vi "Remove newlines from comments.vi"(11 "Comments IN":string caption="Comments") -> (3 "Comments OUT":string caption="Comments")   [LabVIEW 2010]
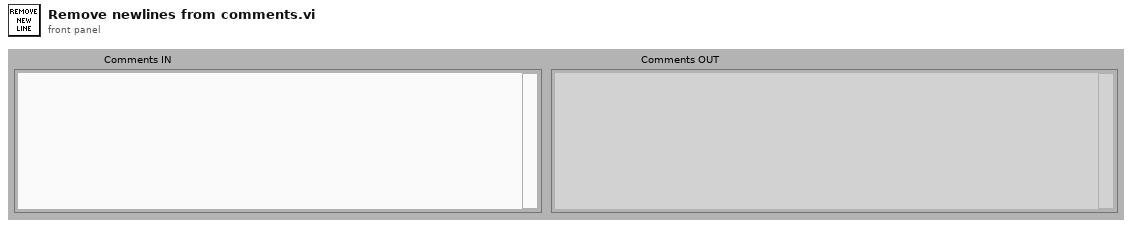
[diagram p1: front panel]
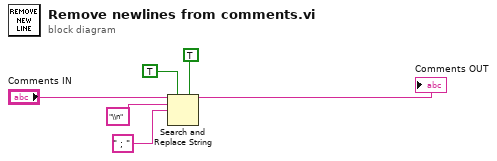
[diagram p0: block diagram]
diagram:
  n1 = Search and Replace String(replace all?=TRUE ("replace all? (F)"), multiline?=TRUE ("multiline? (F)"), input string="Comments IN", search string="\\n", replace string=" ; " ("replace string (\"\")")) -> (result string=→"Comments OUT":string)  [unwired: 3 in, 3 out]
